vi "Update Relay State Model.vi"(7 "position":T1 items=["Open"=10, "Closed"=11], 8 "error in (no error)":errorcluster, 10 "relays to open":string[](array[string]), 11 "SLSC Switch in":refnum<class "SLSC Switch.lvclass">) -> (0 "error out":errorcluster, 3 "SLSC Switch out":refnum<class "SLSC Switch.lvclass">)   [LabVIEW 2015, in "SLSC Switch.lvclass"]
uses:
  SLSC Switch.lvclass
  Route Manager/Position.ctl
  SLSC Switch.lvclass/SLSC Switch.ctl
  Route Manager/Route Manager.lvclass
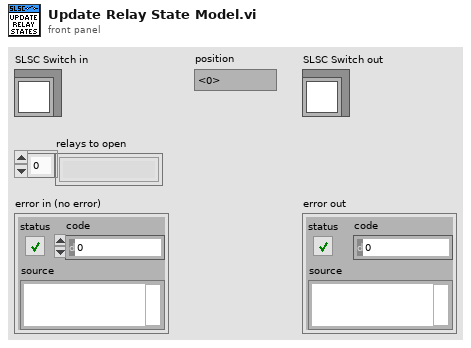
[diagram p1: front panel]
types:
  T1 = typedef "Route Manager.lvclass/Position.ctl" = i32
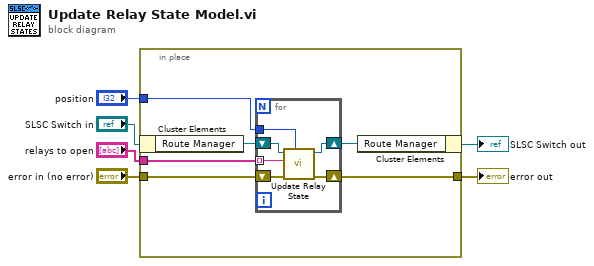
[diagram p0: block diagram]
diagram:
  n1 = in-place {
    in-place-border: "position" -> [w12]
    in-place-border: [w11] -> w5
    in-place-border: "relays to open" -> [w10]
    in-place-border: "error in (no error)" -> [w9]
    n2 = in-place-cluster #1("SLSC Switch in") -> ("Route Manager"=w8:refnum<class "Route Manager.lvclass">)
    n3 = for {
      shift-right: [w16] -> w7
      shift-left: w8 -> [w18]
      shift-right: [w15] -> w11
      shift-left: w9 -> [w17]
      tunnel: w10 -> [w14] mode=indexing
      tunnel: w12 -> [w13]
      n4 = call "Update Relay State.vi"("position"=w13, "error in (no error)"=w17, "relay string"=w14, "Route Manager in"=w18) -> ("error out"=w15:errorcluster, "Route Manager out"=w16:refnum<class "Route Manager.lvclass">)  [unwired: 6 in]
    }
    n5 = in-place-cluster #1("Route Manager"=w7) -> (→"SLSC Switch out":refnum<class "SLSC Switch.lvclass">)
  }
  "error out" <- w5
